vi "GetMasterDeviceAddress_8742.vi"(4 "error in (no error)":errorcluster, 6 "DeviceKey In":string, 7 "CmdLib In":refnum<k24>) -> (0 "error out":errorcluster, 1 "Device Address":i32, 2 "DeviceKey Out":string, 3 "CmdLib Out":refnum<k24>)   [LabVIEW 2009]
uses:
  C:/Code/Apps/Utilities/Picomotor/PicomotorApp/Install/Samples/LabVIEW/Mixed Devices/LabVIEW 2009/CmdLib8742.dll
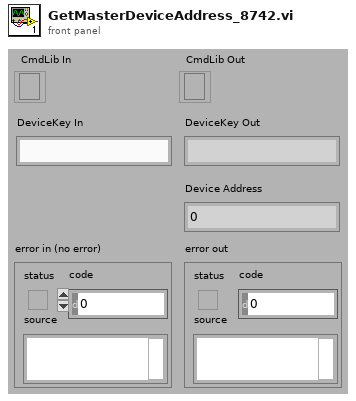
[diagram p1: front panel]
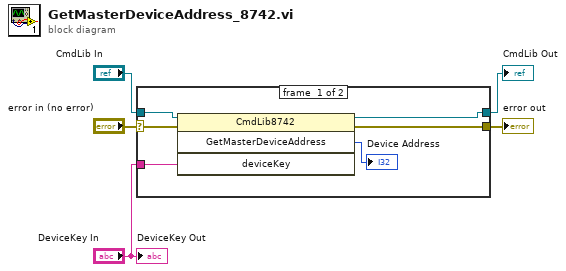
[diagram p0: block diagram]
diagram:
  n1 = case shown="No Error" "error in (no error)" {
    selector: "error in (no error)" -> [w8 w13]
    tunnel: "CmdLib In" -> [w11 w12]
    tunnel: [w10 w12] -> w4
    tunnel: "DeviceKey In" -> [w9 _]
    tunnel: [w7 w13] -> w1
    frame #0 {
      n2 = invoke class="CmdLib8742" method="GetMasterDeviceAddress"(reference=w11, error in=w8, "deviceKey"=w9) -> (reference out=w10:refnum<k24>, error out=w7:errorcluster, "GetMasterDeviceAddress"=→"Device Address":i32)  [unwired: 1 in, 1 out]
    }
    frame #1 {
    }
  }
  "CmdLib Out" <- w4
  "error out" <- w1
  "DeviceKey Out" <- "DeviceKey In"
